vi "RSNRPZ Set Auxiliary Value.vi"(8 "error in (no error)":errorcluster, 9 "Auxiliary Value (0: None)":i32(ring) items=["None", "Min Max", "Rnd Max"], 10 "Channel (1)":i32=1, 11 "VISA session":refnum<visa-resource-name> caption="VISA resource name") -> (0 "error out":errorcluster, 3 "dup VISA session":refnum<visa-resource-name> caption="VISA resource name")   [LabVIEW 2010]
doc: "This VI selects which measurement results are to be made available in the Trace mode.\n\nNote(s):\n\n(1) This VIs is available only for NRP-Z81\n\nRemote-control command(s):\nSENSe:AUXiliary NONE | MINMAX | RNDMAX"
uses:
  rsnrpz_32.dll
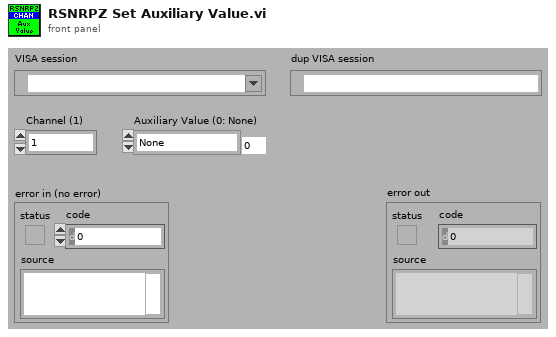
[diagram p1: front panel]
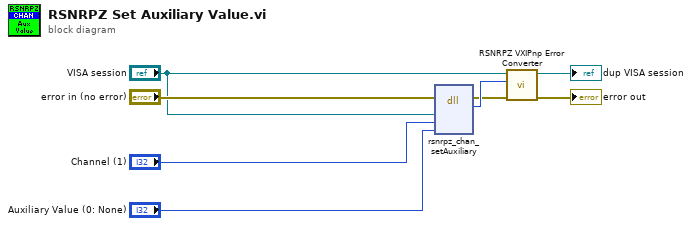
[diagram p0: block diagram]
diagram:
  n1 = dll-call lib="rsnrpz_32.dll" fn="rsnrpz_chan_setAuxiliary"(error in="error in (no error)", "Instrument Handle"="VISA session", "Channel"="Channel (1)", "Auxiliary Value"="Auxiliary Value (0: None)") -> (error out=w5:errorcluster, "Status"=w8:i32)  [unwired: 5 in, 1 out]
  n2 = call <instrlib>:"RSNRPZ VXIPnp Error Converter.vi"("error in"=w5, "VXIPnp error code"=w8, "VISA session"="VISA session") -> ("error out"=→"error out":errorcluster, "dup VISA session"=→"dup VISA session":refnum<visa-resource-name>)  [unwired: 7 in]
